vi "Untitled 1.vi"() -> ()   [LabVIEW 2016]
uses:
  Event Source Messages/Event Generated Msg/Event Generated Msg.lvclass
  Example Sink Messages/Update Array Msg/Update Array Msg.lvclass
  Alternative Example Sink.lvclass
panel:
  out "error out":errorcluster
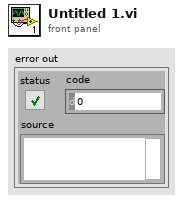
[diagram p1: front panel]
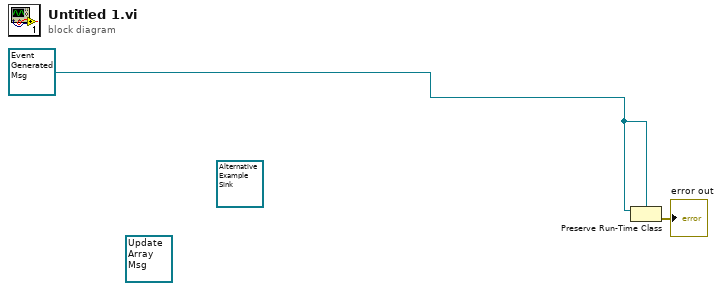
[diagram p0: block diagram]
diagram:
  (unwired) refnum<class "Alternative Example Sink.lvclass"> refnum ("Alternative Example Sink.lvlib:Alternative Example Sink.lvclass")
  (unwired) refnum<class "Update Array Msg.lvclass"> refnum ("Alternative Example Sink.lvlib:Update Array Msg.lvclass")
  w1 = refnum<class "Event Generated Msg.lvclass"> refnum ("Source Event Fire Handler")
  n1 = Preserve Run-Time Class(object in=w1, 2:w1) -> (error out=→"error out":errorcluster)  [unwired: 1 in, 1 out]
